vi "temp_data.vi"(8 "error in (no error)":errorcluster, 11 "TempProbe in":refnum<class "TempProbe.lvclass">) -> (0 "error out":errorcluster, 3 "TempProbe out":refnum<class "TempProbe.lvclass">)   [LabVIEW 2010, in "TempProbe.lvclass"]
uses:
  TempProbe.lvclass
  <vilib>/Analysis/NI_AALBase.lvlib
panel:
  out "temperature":dbl
  out "resistance standard deviation":dbl
  out "resistance average":dbl
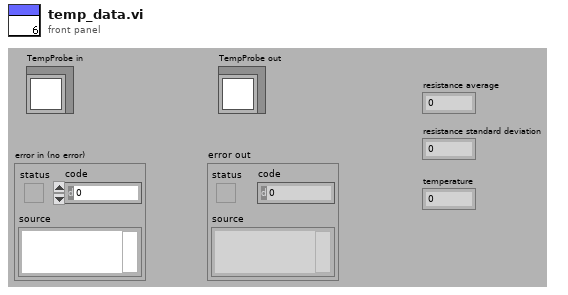
[diagram p1: front panel]
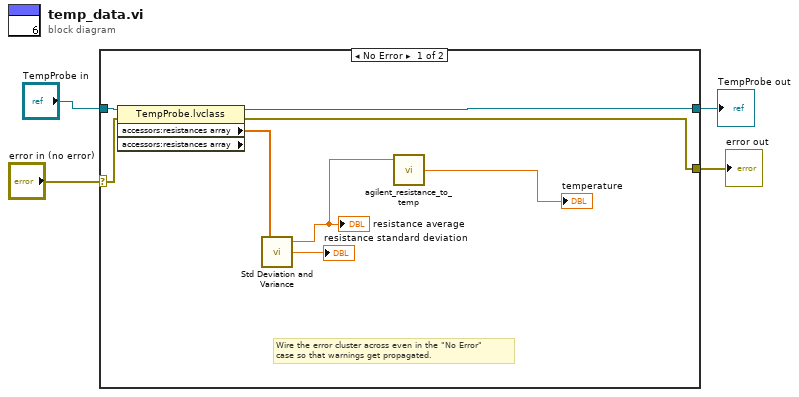
[diagram p0: block diagram]
diagram:
  n1 = case shown="No Error" "error in (no error)" {
    selector: "error in (no error)" -> [w6 w14]
    tunnel: [w5 w14] -> w3
    tunnel: [w11 w13] -> w1
    tunnel: "TempProbe in" -> [w12 w13]
    frame No Error {
      # "Wire the error cluster across even in the \"No Error\"\ncase so that warnings get propagated."
      n2 = property class="TempProbe.lvclass" props=["accessors:resistances array", "accessors:resistances array"](reference=w12, error in=w6) -> (reference out=w11:refnum<class "TempProbe.lvclass">, error out=w5:errorcluster, "accessors:resistances array"=w10:dbl[])  [unwired: 1 out]
      n3 = call <vilib>:"Std Deviation and Variance.vi"("X"=w10) -> ("mean"=w8:dbl, "standard deviation"=→"resistance standard deviation":dbl)  [unwired: 1 in, 1 out]
      "resistance average" <- w8
      n4 = call "agilent_resistance_to_temp.vi"("Resistance"=w8) -> ("Temperature"=→"temperature":dbl)  [unwired: 2 in]
    }
    frame Error {
    }
  }
  "error out" <- w3
  "TempProbe out" <- w1
